vi "dfd_Get String Between Two Strings.vi"(9 "End String":string, 10 "Begin String":string, 11 "Source String":string) -> (3 "Output String":string)   [LabVIEW 2017, in "NI_DigFilterLicensed.lvlib"]
uses:
  <vilib>/addons/Digital Filter Design/NI_DigFilterLicensed.lvlib
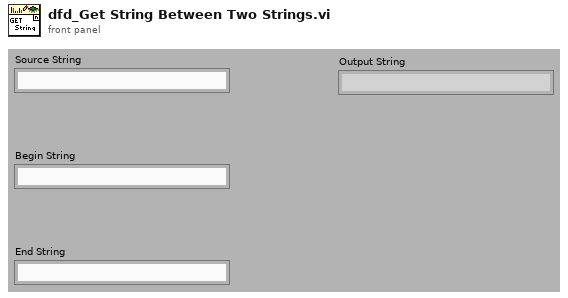
[diagram p1: front panel]
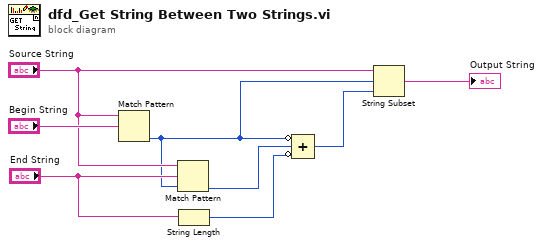
[diagram p0: block diagram]
diagram:
  n1 = Match Pattern(string="Source String", regular expression="Begin String") -> (offset past match=w1:i32)  [unwired: 4 out]
  n2 = Match Pattern(string="Source String", regular expression="End String", offset (0)=w1) -> (offset past match=w5:i32)  [unwired: 3 out]
  n3 = String Length(string="End String") -> (length=w4:i32)
  n4 = Compound Arithmetic op=ADD(invert w1, w5, invert w4) -> (w3:i32)
  n5 = String Subset(string="Source String", offset (0)=w1, length (rest)=w3) -> (substring=→"Output String":string)
